vi "Initialize.vi"(0 "VISA resource name":refnum<visa-resource-name>, 5 "ID Query (T: Check)":bool=TRUE, 7 "Reset (T: Reset)":bool=TRUE, 11 "error in (no error)":errorcluster) -> (4 "VISA resource name out":refnum<visa-resource-name>, 15 "error out":errorcluster {"code" format="%.0x"})   [LabVIEW 2016, in "Fluke 5XXX Series Multicalibrators.lvlib"]
doc: "This VI passes the addressing information in the instrument decriptor to the Instr Open VI and returns the instrument ID. You can optionally reset the instrument by setting the front panel reset control. You must run this VI before using any of the instrument driver VIs for this instrument."
uses:
  Fluke 5XXX Series Multicalibrators.lvlib
panel:
  # "(c) 2005-2012 National Instruments.  ALL RIGHTS RESERVED."
  # "Check\nDon't Check"
  # "Reset\nDon't Reset"
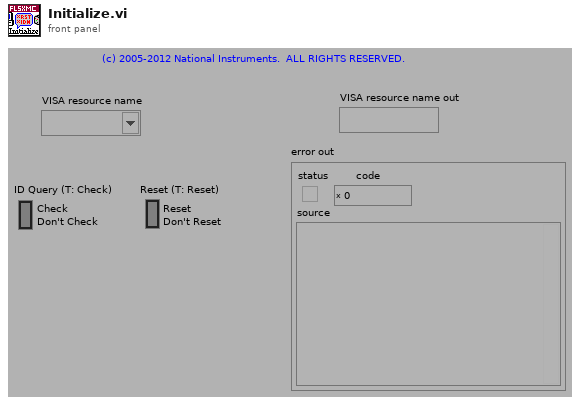
[diagram p1: front panel]
types:
  T1 = cluster{"Status":bool, "Code":i32, "Source (VI Name)":string}
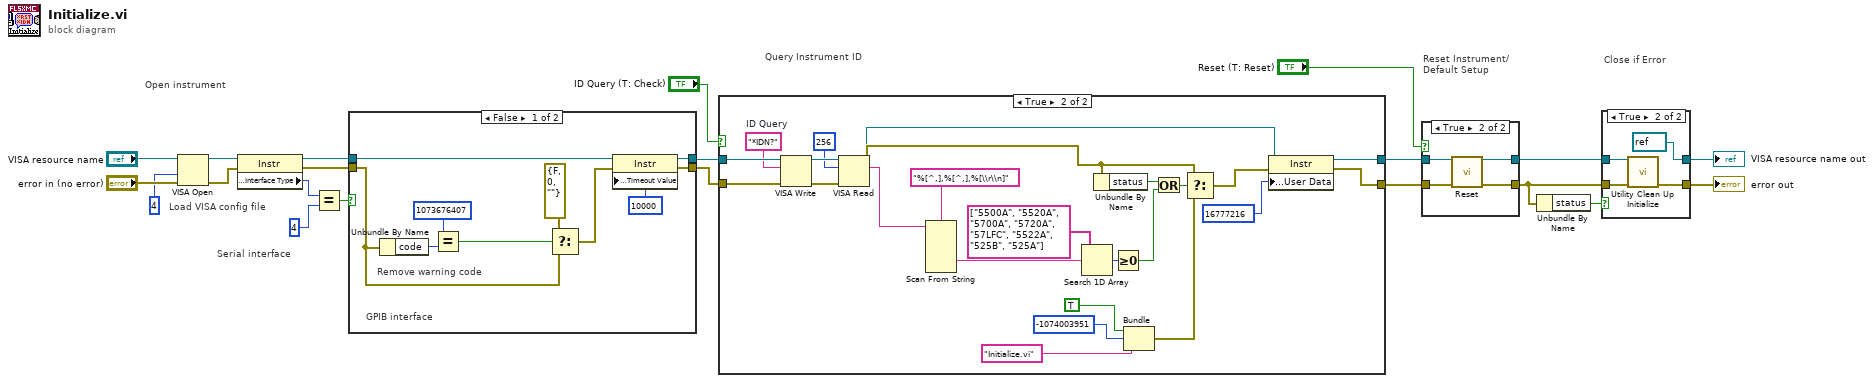
[diagram p0: block diagram]
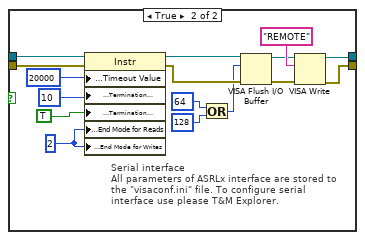
[diagram p2: hidden frame]
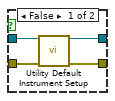
[diagram p4: hidden frame]
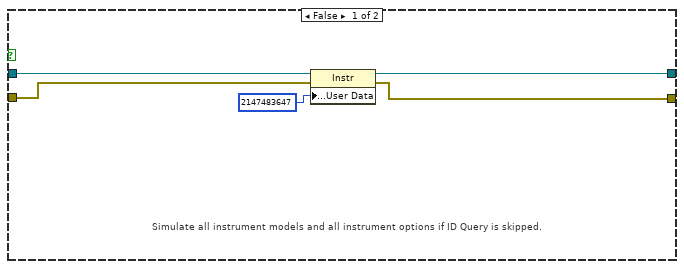
[diagram p5: hidden frame]
diagram:
  # "Serial interface"
  # "Load VISA config file"
  # "Close if Error"
  # "Query Instrument ID"
  # "Reset Instrument/\nDefault Setup"
  # "Open instrument"
  n1 = VISA Open(access mode=u32 4, error in (no error)="error in (no error)", VISA resource name="VISA resource name") -> (VISA resource name=w12:refnum<visa-resource-name>, error out=w11:errorcluster)  [unwired: 2 in]
  n2 = property on="Property Node" class="Instr"(reference=w12, error in=w11) -> (reference out=w7:refnum<visa-resource-name>, error out=w8:errorcluster, "Interface Information:Interface Type"=w10:u16)
  n3 = Equal?(x=w10, y=u16 4) -> (x = y?=w9:bool)
  n4 = case shown="False" w9 {
    tunnel: w8 -> [w23 w46]
    tunnel: w7 -> [w31 w47]
    tunnel: [w30 w38] -> w3
    tunnel: [w29 w35] -> w2
    frame False {
      # "Remove warning code"
      # "GPIB interface"
      n5 = Unbundle By Name(w23) -> ("code"=w24:i32)
      n6 = Equal?(x=1073676407, y=w24) -> (x = y?=w26:bool)
      n7 = Select(t=errorcluster {"status"=FALSE, "code"=0, "source"=""} ("error out"), s=w26, f=w23) -> (s? t:f=w22:errorcluster)
      n8 = property on="Property Node" class="Instr"(reference=w31, error in=w22, "General Settings:Timeout Value"=u32 10000 ("Tmo Value")) -> (reference out=w29:refnum<visa-resource-name>, error out=w30:errorcluster)
    }
    frame True {
      w42 = u16 2 ("ASRL End In")
      # "Serial interface\nAll parameters of ASRLx interface are stored to the \"visaconf.ini\" file. To configure serial interface use please T&M Explorer."
      n9 = property on="Property Node" class="Instr"(reference=w47, error in=w46, "General Settings:Timeout Value"=u32 20000, "Message Based Settings:Termination Character"=u8 10 ("TermChar"), "Message Based Settings:Termination Character Enable"=TRUE ("TermChar En"), "Serial Settings:End Mode for Reads"=w42, "Serial Settings:End Mode for Writes"=w42) -> (reference out=w41:refnum<visa-resource-name>, error out=w40:errorcluster)
      n10 = Or(x=u32 64, y=u32 128) -> (x .or. y?=w32:u32)
      n11 = VISA Flush I/O Buffer(VISA resource name=w41, mask (16)=w32, error in (no error)=w40) -> (VISA resource name out=w36:refnum<visa-resource-name>, error out=w37:errorcluster)
      n12 = VISA Write(VISA resource name=w36, write buffer="REMOTE" ("ID Query"), error in (no error)=w37) -> (VISA resource name out=w35:refnum<visa-resource-name>, error out=w38:errorcluster)  [unwired: 1 out]
    }
  }
  n13 = case shown="True" "ID Query (T: Check)" {
    tunnel: [w51 w57] -> w20
    tunnel: [w52 w59] -> w21
    tunnel: w2 -> [w49 w75]
    tunnel: w3 -> [w50 w76]
    frame False {
      # "Simulate all instrument models and all instrument options if ID Query is skipped."
      n14 = property on="Property Node" class="Instr"(reference=w49, error in=w50, "General Settings:User Data"=u32 2147483647 ("y")) -> (reference out=w52:refnum<visa-resource-name>, error out=w51:errorcluster)
    }
    frame True {
      w66 = "*IDN?"  # ID Query
      n15 = VISA Write(VISA resource name=w75, write buffer=w66, error in (no error)=w76) -> (VISA resource name out=w72:refnum<visa-resource-name>, error out=w70:errorcluster)  [unwired: 1 out]
      n16 = VISA Read(VISA resource name=w72, byte count=u32 256, error in (no error)=w70) -> (VISA resource name out=w60:refnum<visa-resource-name>, read buffer=w61:string, error out=w71:errorcluster)  [unwired: 1 out]
      n17 = Scan From String(format string="%[^,],%[^,],%[\\r\\n]" ("Format String"), input string=w61) -> (output 2=w54:string)  [unwired: 7 in, 3 out]
      n18 = Search 1D Array(1D array=string[] ["5500A", "5520A", "5700A", "5720A", "57LFC", "5522A", "525B", "525A"] ("Array Constant"), element=w54) -> (index of element=w53:i32)  [unwired: 1 in]
      n19 = Unbundle By Name(w71) -> ("status"=w68:bool)
      n20 = Greater Or Equal To 0?(x=w53) -> (x >= 0?=w73:bool)
      n21 = Bundle("Status"=TRUE, "Code"=-1074003951, "Source (VI Name)"="Initialize.vi") -> (w65:T1)  [unwired: 1 in]
      n22 = Or(x=w68, y=w73) -> (x .or. y?=w69:bool)
      n23 = Select(t=w71, s=w69, f=w65) -> (s? t:f=w58:T1)
      n24 = property on="Property Node" class="Instr"(reference=w60, error in=w58, "General Settings:User Data"=u32 16777216) -> (reference out=w59:refnum<visa-resource-name>, error out=w57:errorcluster)
    }
  }
  n25 = case shown="True" "Reset (T: Reset)" {
    tunnel: w20 -> [w79 w81]
    tunnel: [w78 w84] -> w16
    tunnel: w21 -> [w80 w82]
    tunnel: [w77 w83] -> w15
    frame False {
      n26 = call "Utility Default Instrument Setup.vi"("VISA resource name"=w80, "error in (no error)"=w79) -> ("VISA resource name out"=w77:refnum<visa-resource-name>, "error out"=w78:errorcluster)  [unwired: 12 in]
    }
    frame True {
      n27 = call "Reset.vi"("VISA resource name"=w82, "error in (no error)"=w81) -> ("VISA resource name out"=w83:refnum<visa-resource-name>, "error out"=w84:errorcluster)  [unwired: 12 in]
    }
  }
  n28 = Unbundle By Name(w16) -> ("status"=w17:bool)
  n29 = case shown="True" w17 {
    tunnel: w15 -> [w86 w90]
    tunnel: w16 -> [w85 w89]
    tunnel: [w86 refnum<visa-resource-name> refnum ("VISA resource name out")] -> w14
    tunnel: [w85 w88] -> w13
    frame False {
    }
    frame True {
      n30 = call "Utility Clean Up Initialize.vi"("VISA session"=w90, "error in (no error)"=w89) -> ("error out"=w88:errorcluster)  [unwired: 13 in]
    }
  }
  "VISA resource name out" <- w14
  "error out" <- w13
